vi "Publis Y Axis.vi"(11 "Y Axis":T1) -> ()   [LabVIEW 2017]
uses:
  <vilib>/Rock Robotics/Network Tables/NT Write Number.vi
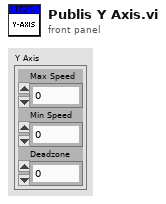
[diagram p1: front panel]
types:
  T1 = cluster{"Max Speed":dbl, "Min Speed":dbl, "Deadzone":dbl}
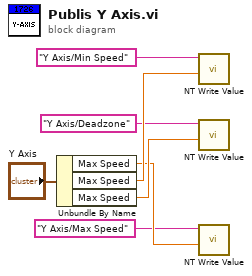
[diagram p0: block diagram]
diagram:
  n1 = Unbundle By Name("Y Axis") -> ("Max Speed"=w5:dbl, "Max Speed"=w6:dbl, "Max Speed"=w7:dbl)
  n2 = call-poly <vilib>:"NT Write Value.vi"("Numeric"=w6, "Name"="Y Axis/Min Speed") -> ()  [unwired: 9 in, 1 out]
  n3 = call-poly <vilib>:"NT Write Value.vi"("Numeric"=w7, "Name"="Y Axis/Deadzone") -> ()  [unwired: 9 in, 1 out]
  n4 = call-poly <vilib>:"NT Write Value.vi"("Numeric"=w5, "Name"="Y Axis/Max Speed") -> ()  [unwired: 9 in, 1 out]
